vi "Is Value Type Valid.vi"(8 "error in (no error)":errorcluster, 10 "Value Type to Check":string, 11 "DriverSetting in":refnum<class "DriverSetting.lvclass">) -> (0 "error out":errorcluster, 2 "Is Valid":bool, 3 "DriverSetting out":refnum<class "DriverSetting.lvclass">)   [LabVIEW 2023, in "HAF.lvlib" / "DriverSetting.lvclass"]
uses:
  DriverSetting.lvclass
  Valid Data Types.ctl
  DriverSetting.lvclass/DriverSetting.ctl
  <vilib>/Utility/error.llb/Trim Whitespace One-Sided.vi
  HAF.lvlib
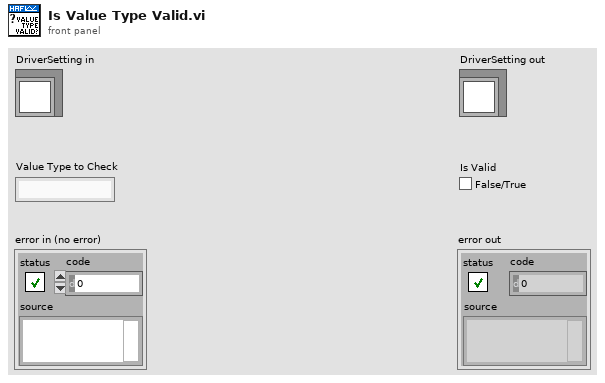
[diagram p1: front panel]
types:
  T1 = typedef "HAF.lvlib/Valid Data Types.ctl" = cluster{"U8":string, "U16":string, "U32":string, "U64":string, "I8":string, "I16 ":string, "I32":string, "I64":string, "SGL":string, "DBL":string, "String":string, "Boolean":string}
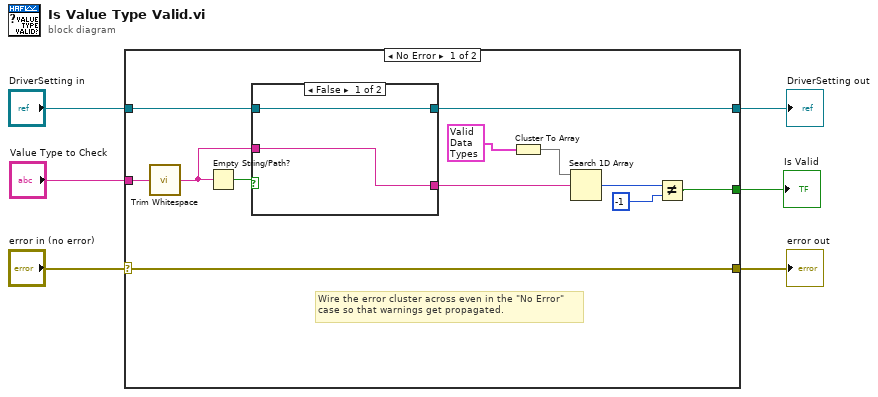
[diagram p0: block diagram]
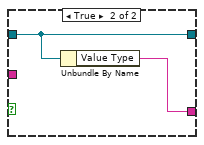
[diagram p2: hidden frame]
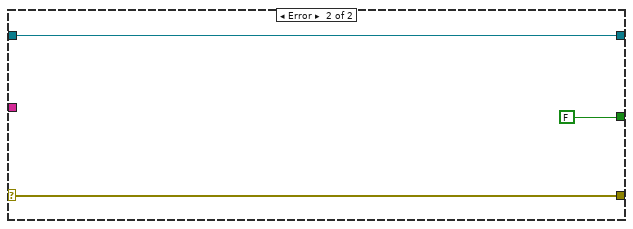
[diagram p3: hidden frame]
diagram:
  n1 = case shown="No Error" "error in (no error)" {
    selector: "error in (no error)" -> [w18 w25]
    tunnel: [w18 w25] -> w5
    tunnel: [w16 w24] -> w3
    tunnel: "DriverSetting in" -> [w17 w24]
    tunnel: "Value Type to Check" -> [w15 _]
    tunnel: [w8 FALSE] -> w1
    frame No Error {
      # "Wire the error cluster across even in the \"No Error\"\ncase so that warnings get propagated."
      n2 = call <vilib>:"Trim Whitespace.vi"("string"=w15) -> ("trimmed string"=w13:string)  [unwired: 1 in]
      n3 = Empty String/Path?(string/path=w13) -> (empty?=w14:bool)
      n4 = case shown="False" w14 {
        tunnel: w17 -> [w20 w21]
        tunnel: [w20 w21] -> w16
        tunnel: w13 -> [w19 _]
        tunnel: [w19 w22] -> w11
        frame False {
        }
        frame True {
          n5 = Unbundle By Name(w21) -> ("Value Type"=w22:string)
        }
      }
      n6 = Cluster To Array(cluster=T1 {"U8"="U8", "U16"="U16", "U32"="U32", "U64"="U64", "I8"="I8", "I16 "="I16", "I32"="I32", "I64"="I64", "SGL"="SGL", "DBL"="DBL", "String"="String", "Boolean"="Boolean"} ("Valid Data Types")) -> (array=w12:string[])
      n7 = Search 1D Array(1D array=w12, element=w11) -> (index of element=w10:i32)  [unwired: 1 in]
      n8 = Not Equal?(x=w10, y=-1) -> (x != y?=w8:bool)
    }
    frame Error {
    }
  }
  "error out" <- w5
  "DriverSetting out" <- w3
  "Is Valid" <- w1
